vi "Initialize System (Std 2011).vi"(0 "CFG-1":T8={"PMU ID"=1, "time base"=10000000, "nominal frequency"=enum."60 Hz", "reporting rate [fps]"=60, "station name"="", "data format"=15, "phasor channels"=[], "analog channels"=[], "digital channels"=[]} {"digital channels"."digital unit" format="%08x"; "analog channels"."analog unit" format="%08x"; "phasor channels"."phasor unit scaling" max=16777215 format="%06x"; "phasor channels"."phasor unit" items=["Voltage [V]"=0, "Current [A]"=16777216]; "data format" format="%016b"}, 1 "physical channels":T11[](array[typedef]), 2 "performance class":enum8{"M Class", "P Class"}(ring), 5 "CFG-2":T8={"PMU ID"=1, "time base"=10000000, "nominal frequency"=enum."60 Hz", "reporting rate [fps]"=60, "station name"="", "data format"=15, "phasor channels"=[], "analog channels"=[], "digital channels"=[]} {"digital channels"."digital unit" format="%08x"; "analog channels"."analog unit" format="%08x"; "phasor channels"."phasor unit scaling" max=16777215 format="%06x"; "phasor channels"."phasor unit" items=["Voltage [V]"=0, "Current [A]"=16777216]; "data format" format="%016b"}, 7 "CFG-3":T3={"PMU ID"=1, "global PMU ID"=1, "time base"=10000000, "nominal frequency"=enum."60 Hz", "reporting rate [fps]"=60, "station name"="", "data format"=15, "phasor channels"=[], "analog channels"=[], "digital channels"=[]} {"data format" format="%016b"; "phasor channels"."phasor unit" items=["Voltage [V]"=0, "Current [A]"=16777216]; "phasor channels"."data modification flag" format="%016b"; "digital channels"."digital unit" format="%08x"}, 9 "header":string, 11 "error in (no error)":errorcluster, 12 "configuration for data frame":T2) -> (4 "initial samples to read":u32=250, 6 "M Class memory information":T7, 8 "algorithm factors [us]":T1, 10 "system info out":refnum<class "PMU System Info.lvclass">, 15 "error out":errorcluster)   [LabVIEW 2014, in "NI_EP_PMU.lvlib"]
doc: "Sets the configuration for a phasor measurement unit (PMU) system as defined in IEEE Std C37.118.1-2011 and IEEE Std C37.118.2-2011."
uses:
  <vilib>/addons/Electrical Power/PMU/NI_EP_PMU.lvlib
  <vilib>/addons/Electrical Power/PMU/Common/Classes/PMU System Info/PMU System Info.lvclass
  <vilib>/addons/Electrical Power/PMU/Common/Controls/pmu_CFG Input.ctl
  <vilib>/addons/Electrical Power/PMU/Common/Controls/pmu_Phasor Channel.ctl
  <vilib>/addons/Electrical Power/PMU/Common/Controls/pmu_Analog Channel.ctl
  <vilib>/addons/Electrical Power/PMU/Common/Controls/pmu_Digital Channel.ctl
  <vilib>/addons/Electrical Power/PMU/Common/Controls/pmu_Physical Channel.ctl
  <vilib>/addons/Electrical Power/PMU/Common/Controls/pmu_Channel Phase.ctl
  <vilib>/addons/Electrical Power/PMU/Common/Controls/pmu_M Class Memory Information.ctl
  <vilib>/addons/Electrical Power/PMU/Common/Controls/pmu_CFG-3 Input.ctl
  <vilib>/addons/Electrical Power/PMU/Common/Controls/pmu_CFG-3 Phasor Channels.ctl
  <vilib>/addons/Electrical Power/PMU/Common/Controls/pmu_CFG-3 Analog Channels.ctl
  <vilib>/addons/Electrical Power/PMU/Common/Controls/pmu_CFG for Data Frame.ctl
  <vilib>/addons/Electrical Power/PMU/Common/Controls/pmu_CFG-3 Dynamic Response Factors.ctl
  <vilib>/addons/Electrical Power/PMU/Common/Controls/pmu_Frequency Detector Settings.ctl
  <vilib>/addons/Electrical Power/PMU/Common/Controls/pmu_ROCOF Detector Settings.ctl
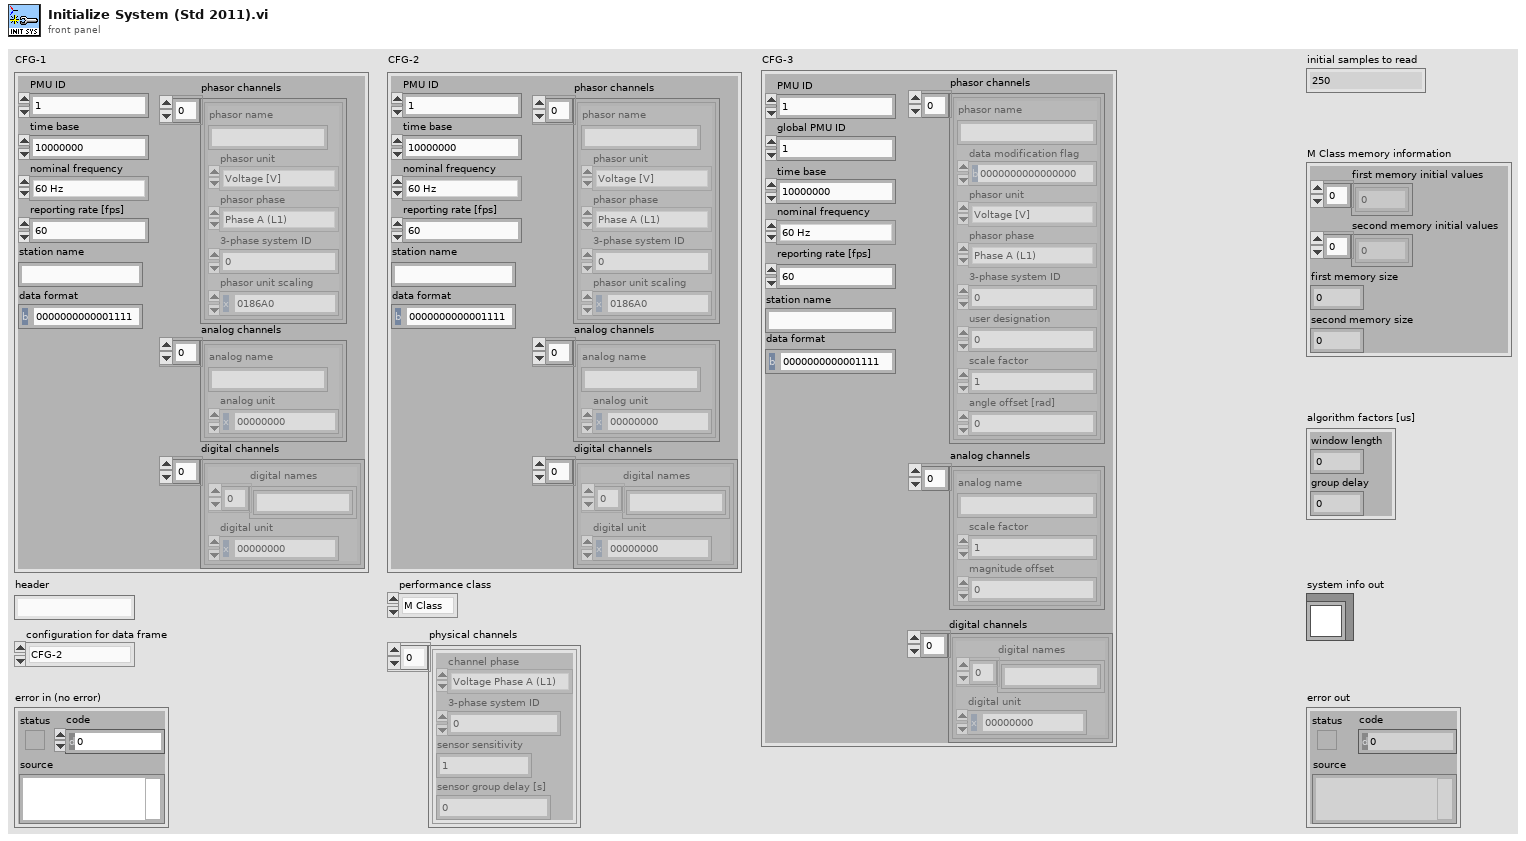
[diagram p1: front panel]
types:
  T1 = typedef "NI_EP_PMU.lvlib/pmu_CFG-3 Dynamic Response Factors.ctl" = cluster{"window length":i32, "group delay":i32}
  T2 = typedef "NI_EP_PMU.lvlib/pmu_CFG for Data Frame.ctl" = enum8{"CFG-2", "CFG-3"}
  T3 = typedef "NI_EP_PMU.lvlib/pmu_CFG-3 Input.ctl" = cluster{"PMU ID":u16, "global PMU ID":u64, "time base":u32, "nominal frequency":enum16{"50 Hz", "60 Hz"}, "reporting rate [fps]":i16, "station name":string, "data format":u16, "phasor channels":T4[], "analog channels":T5[], "digital channels":T6[]}
  T4 = typedef "NI_EP_PMU.lvlib/pmu_CFG-3 Phasor Channels.ctl" = cluster{"phasor name":string, "data modification flag":u16, "phasor unit":u32, "phasor phase":enum16{"Phase A (L1)", "Phase B (L2)", "Phase C (L3)", "Phase N", "Positive sequence", "Negative sequence", "Zero sequence"}, "3-phase system ID":u8, "user designation":u8, "scale factor":sgl, "angle offset [rad]":sgl}
  T5 = typedef "NI_EP_PMU.lvlib/pmu_CFG-3 Analog Channels.ctl" = cluster{"analog name":string, "scale factor":sgl, "magnitude offset":sgl}
  T6 = typedef "NI_EP_PMU.lvlib/pmu_Digital Channel.ctl" = cluster{"digital names":string[], "digital unit":u32}
  T7 = typedef "NI_EP_PMU.lvlib/pmu_M Class Memory Information.ctl" = cluster{"first memory initial values":fxp<+/-,18,-4>[], "second memory initial values":fxp<+/-,19,-3>[], "first memory size":u32, "second memory size":u32}
  T8 = typedef "NI_EP_PMU.lvlib/pmu_CFG Input.ctl" = cluster{"PMU ID":u16, "time base":u32, "nominal frequency":enum16{"50 Hz", "60 Hz"}, "reporting rate [fps]":i16, "station name":string, "data format":u16, "phasor channels":T9[], "analog channels":T10[], "digital channels":T6[]}
  T9 = typedef "NI_EP_PMU.lvlib/pmu_Phasor Channel.ctl" = cluster{"phasor name":string, "phasor unit":u32, "phasor phase":enum16{"Phase A (L1)", "Phase B (L2)", "Phase C (L3)", "Phase N", "Positive sequence", "Negative sequence", "Zero sequence"}, "3-phase system ID":u8, "phasor unit scaling":u32}
  T10 = typedef "NI_EP_PMU.lvlib/pmu_Analog Channel.ctl" = cluster{"analog name":string, "analog unit":u32}
  T11 = typedef "NI_EP_PMU.lvlib/pmu_Physical Channel.ctl" = cluster{"channel phase":T12, "3-phase system ID":u8, "sensor sensitivity":dbl, "sensor group delay [s]":dbl}
  T12 = typedef "NI_EP_PMU.lvlib/pmu_Channel Phase.ctl" = enum16{"Voltage Phase A (L1)", "Voltage Phase B (L2)", "Voltage Phase C (L3)", "Voltage Phase N (Neutral)", "Current Phase A (L1)", "Current Phase B (L2)", "Current Phase C (L3)", "Current Phase N (Neutral)", "Voltage Phase AB (L1L2)", "Voltage Phase BC (L2L3)", "Voltage Phase CA (L3L1)"}
  T13 = typedef "NI_EP_PMU.lvlib/pmu_ROCOF Detector Settings.ctl" = cluster{"ROCOF window width":i32}
  T14 = typedef "NI_EP_PMU.lvlib/pmu_Frequency Detector Settings.ctl" = cluster{"frequency window width":i32}
  T15 = cluster{"3-phase system ID":u8, "channel phase":T12}[]
  T16 = typedef "NI_EP_PMU.lvlib/pmu_Phasor Channel Info.ctl" = cluster{"channel indexes":i32[], "phasor phase":enum16{"Phase A (L1)", "Phase B (L2)", "Phase C (L3)", "Phase N", "Positive sequence", "Negative sequence", "Zero sequence"}, "connection type":T17}
  T17 = typedef "NI_EP_PMU.lvlib/pmu_Connection Type.ctl" = enum16{"Wye", "Delta"}
  T18 = typedef "NI_EP_PMU.lvlib/pmu_CFG Class.ctl" = cluster{"station name":string, "PMU ID":u16, "time base":u32, "nominal frequency":enum16{"50 Hz", "60 Hz"}, "reporting rate":i16, "phasor number":u16, "analog number":u16, "digital number":u16, "channel names":string[], "phasor units":u32[], "analog units":u32[], "digital units":u32[], "data format":u16, "number of PMUs":u16}
  T19 = typedef "NI_EP_PMU.lvlib/pmu_CFG-3 Class.ctl" = cluster{"station name":string, "PMU ID":u16, "global PMU ID":u64, "time base":u32, "nominal frequency":enum16{"50 Hz", "60 Hz"}, "reporting rate":i16, "phasor number":u16, "analog number":u16, "digital number":u16, "channel names":string[], "phasor scale first 4 bytes":u32[], "phasor scale factors":sgl[], "phasor angle offsets [rad]":sgl[], "analog scale factors":sgl[], "analog magnitude offsets":sgl[], "digital units":u32[], "data format":u16, "number of PMUs":u16}
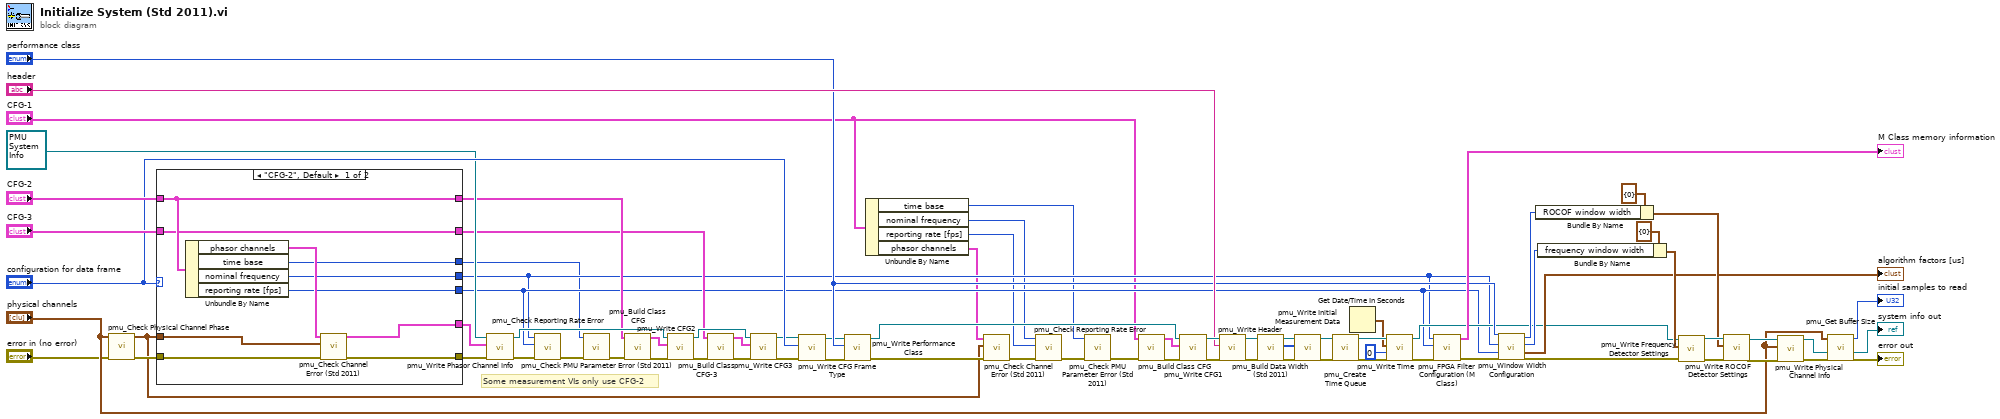
[diagram p0: block diagram]
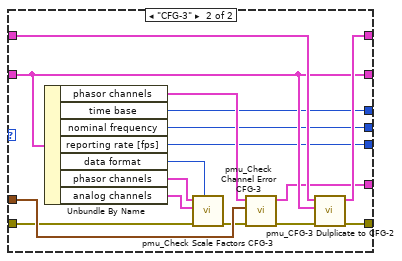
[diagram p2: hidden frame]
diagram:
  # "Some measurement VIs only use CFG-2"
  n1 = call <vilib>:"pmu_Check Physical Channel Phase.vi"("error in (no error)"="error in (no error)", "physical channels in"="physical channels") -> ("error out"=w12:errorcluster, "physical channel out"=w6:T15)  [unwired: 8 in]
  n2 = case shown="\"CFG-2\", Default" "configuration for data frame" {
    tunnel: w12 -> [w82 w88]
    tunnel: "CFG-2" -> [w84 w102]
    tunnel: w6 -> [w80 w95]
    tunnel: "CFG-3" -> [w83 w99]
    tunnel: [w83 w99] -> w23
    tunnel: [w84 w100] -> w24
    tunnel: [w79 w94] -> w26
    tunnel: [w78 w101] -> w20
    tunnel: [w86 w98] -> w17
    tunnel: [w85 w97] -> w18
    tunnel: [w81 w96] -> w16
    frame "CFG-2", Default {
      n3 = Unbundle By Name(w84) -> ("phasor channels"=w87:T9[], "time base"=w81:u32, "nominal frequency"=w86:enum16{"50 Hz", "60 Hz"}, "reporting rate [fps]"=w85:i16)
      n4 = call <vilib>:"pmu_Check Channel Error (Std 2011).vi"("error in (no error)"=w82, "physical channel in"=w80, "phasor channels"=w87) -> ("error out"=w78:errorcluster, "phasor channel info"=w79:T16[])  [unwired: 7 in]
    }
    frame "CFG-3" {
      n5 = Unbundle By Name(w99) -> ("phasor channels"=w103:T4[], "time base"=w96:u32, "nominal frequency"=w98:enum16{"50 Hz", "60 Hz"}, "reporting rate [fps]"=w97:i16, "data format"=w90:u16, "phasor channels"=w92:T4[], "analog channels"=w91:T5[])
      n6 = call <vilib>:"pmu_Check Scale Factors CFG-3.vi"("data format"=w90, "error in (no error)"=w88, "analog channels"=w91, "phasor channels"=w92) -> ("error out"=w89:errorcluster)  [unwired: 7 in]
      n7 = call <vilib>:"pmu_Check Channel Error CFG-3.vi"("error in (no error)"=w89, "physical channel in"=w95, "phasor channels"=w103) -> ("error out"=w93:errorcluster, "phasor channel info"=w94:T16[])  [unwired: 7 in]
      n8 = call <vilib>:"pmu_CFG-3 Dulplicate to CFG-2.vi"("error in (no error)"=w93, "CFG-3"=w99, "CFG-2"=w102) -> ("error out"=w101:errorcluster, "CFG-2 output"=w100:T8)  [unwired: 7 in]
    }
  }
  n9 = call <vilib>:"pmu_Write Phasor Channel Info.vi"("error in (no error)"=w20, "phasor channel info"=w26, "system info in"=refnum<class "PMU System Info.lvclass"> refnum ("PMU System Info.lvclass")) -> ("error out"=w19:errorcluster, "system info out"=w29:refnum<class "PMU System Info.lvclass">)  [unwired: 7 in]
  n10 = call <vilib>:"pmu_Check Reporting Rate Error.vi"("error in (no error)"=w19, "reporting rate"=w18, "nominal frequency"=w17) -> ("error out"=w15:errorcluster)  [unwired: 8 in]
  n11 = call <vilib>:"pmu_Check PMU Parameter Error (Std 2011).vi"("error in (no error)"=w15, "time base"=w16) -> ("error out"=w14:errorcluster)  [unwired: 9 in]
  n12 = call <vilib>:"pmu_Build Class CFG.vi"("error in (no error)"=w14, "CFG input"=w24) -> ("error out"=w28:errorcluster, "CFG class"=w27:T18)  [unwired: 8 in]
  n13 = call <vilib>:"pmu_Write CFG2.vi"("error in (no error)"=w28, "CFG-2"=w27, "system info in"=w29) -> ("error out"=w33:errorcluster, "system info out"=w32:refnum<class "PMU System Info.lvclass">)  [unwired: 7 in]
  n14 = call <vilib>:"pmu_Build Class CFG-3.vi"("error in (no error)"=w33, "CFG-3"=w23) -> ("error out"=w30:errorcluster, "CFG-3 class"=w31:T19)  [unwired: 8 in]
  n15 = call <vilib>:"pmu_Write CFG3.vi"("error in (no error)"=w30, "CFG-3 class"=w31, "system info in"=w32) -> ("error out"=w22:errorcluster, "system info out"=w21:refnum<class "PMU System Info.lvclass">)  [unwired: 7 in]
  n16 = call <vilib>:"pmu_Write CFG Frame Type.vi"("error in (no error)"=w22, "configuration frame option"="configuration for data frame", "system info in"=w21) -> ("error out"=w41:errorcluster, "system info out"=w34:refnum<class "PMU System Info.lvclass">)  [unwired: 7 in]
  n17 = call <vilib>:"pmu_Write Performance Class.vi"("error in (no error)"=w41, "performance class"="performance class", "system info in"=w34) -> ("error out"=w7:errorcluster, "system info out"=w44:refnum<class "PMU System Info.lvclass">)  [unwired: 7 in]
  n18 = Unbundle By Name("CFG-1") -> ("time base"=w1:u32, "nominal frequency"=w2:enum16{"50 Hz", "60 Hz"}, "reporting rate [fps]"=w3:i16, "phasor channels"=w4:T9[])
  n19 = call <vilib>:"pmu_Check Channel Error (Std 2011).vi"("error in (no error)"=w7, "physical channel in"=w6, "phasor channels"=w4) -> ("error out"=w10:errorcluster)  [unwired: 7 in, 1 out]
  n20 = call <vilib>:"pmu_Check Reporting Rate Error.vi"("error in (no error)"=w10, "reporting rate"=w3, "nominal frequency"=w2) -> ("error out"=w9:errorcluster)  [unwired: 8 in]
  n21 = call <vilib>:"pmu_Check PMU Parameter Error (Std 2011).vi"("error in (no error)"=w9, "time base"=w1) -> ("error out"=w8:errorcluster)  [unwired: 9 in]
  n22 = call <vilib>:"pmu_Build Class CFG.vi"("error in (no error)"=w8, "CFG input"="CFG-1") -> ("error out"=w74:errorcluster, "CFG class"=w76:T18)  [unwired: 8 in]
  n23 = call <vilib>:"pmu_Write CFG1.vi"("error in (no error)"=w74, "CFG-1"=w76, "system info in"=w44) -> ("error out"=w67:errorcluster, "system info out"=w69:refnum<class "PMU System Info.lvclass">)  [unwired: 7 in]
  n24 = call <vilib>:"pmu_Write Header.vi"("error in (no error)"=w67, "header"="header", "system info in"=w69) -> ("error out"=w66:errorcluster, "system info out"=w68:refnum<class "PMU System Info.lvclass">)  [unwired: 7 in]
  n25 = call <vilib>:"pmu_Build Data Width (Std 2011).vi"("error in (no error)"=w66, "system info in"=w68) -> ("error out"=w70:errorcluster, "init meas data"=w71:u8[], "system info out"=w72:refnum<class "PMU System Info.lvclass">)  [unwired: 7 in]
  n26 = call <vilib>:"pmu_Write Initial Measurement Data.vi"("error in (no error)"=w70, "init meas data"=w71, "system info in"=w72) -> ("error out"=w63:errorcluster, "system info out"=w64:refnum<class "PMU System Info.lvclass">)  [unwired: 7 in]
  n27 = call <vilib>:"pmu_Create Time Queue.vi"("error in (no error)"=w63, "PMU System Info in"=w64) -> ("error out"=w61:errorcluster, "PMU System Info out"=w62:refnum<class "PMU System Info.lvclass">)  [unwired: 8 in]
  n28 = Get Date/Time In Seconds() -> (seconds since 1Jan1904=w60:timestamp)
  n29 = call <vilib>:"pmu_Write Time .vi"("error in (no error)"=w61, "time quality"=u8 0, "time stamp"=w60, "system info in"=w62) -> ("error out"=w39:errorcluster, "system info out"=w36:refnum<class "PMU System Info.lvclass">)  [unwired: 6 in]
  n30 = call <vilib>:"pmu_FPGA Filter Configuration (M Class).vi"("error in (no error)"=w39, "reporting rate"=w18, "nominal frequency"=w17) -> ("error out"=w38:errorcluster, "M Class memory configuration"=→"M Class memory information":T7)  [unwired: 7 in]
  n31 = call <vilib>:"pmu_Window Width Configuration.vi"("error in (no error)"=w38, "reporting rate"=w18, "nominal frequency"=w17, "Performance Class"="performance class") -> ("error out"=w37:errorcluster, "dynamic response factors"=→"algorithm factors [us]":T1, "frequency window width"=w53:i32, "ROCOF window width"=w47:i32)  [unwired: 4 in]
  n32 = Bundle By Name(cluster=T13 {"ROCOF window width"=0} ("ROCOF detector settings"), "ROCOF window width"=w47) -> (w48:T13)
  n33 = Bundle By Name(cluster=T14 {"frequency window width"=0} ("frequency detector settings"), "frequency window width"=w53) -> (w57:T14)
  n34 = call <vilib>:"pmu_Write Frequency Detector Settings.vi"("error in (no error)"=w37, "frequency detector settings"=w57, "system info in"=w36) -> ("error out"=w51:errorcluster, "system info out"=w52:refnum<class "PMU System Info.lvclass">)  [unwired: 7 in]
  n35 = call <vilib>:"pmu_Write ROCOF Detector Settings.vi"("error in (no error)"=w51, "ROCOF detector settings"=w48, "system info in"=w52) -> ("error out"=w50:errorcluster, "system info out"=w46:refnum<class "PMU System Info.lvclass">)  [unwired: 7 in]
  n36 = call <vilib>:"pmu_Write Physical Channel Info.vi"("error in (no error)"=w50, "physical channels"="physical channels", "system info in"=w46) -> ("error out"=w55:errorcluster, "system info out"=w56:refnum<class "PMU System Info.lvclass">)  [unwired: 7 in]
  n37 = call <vilib>:"pmu_Get Buffer Size.vi"("error in (no error)"=w55, "PMU System Info in"=w56, "physical channels"="physical channels") -> ("error out"=→"error out":errorcluster, "PMU System Info out"=→"system info out":refnum<class "PMU System Info.lvclass">, "buffer size (samples)"=→"initial samples to read":u32)  [unwired: 6 in]
